vi "update_counter_entry_small.vi"(8 "error in":errorcluster, 10 "Integer Time":i64, 11 "input cluster":cluster{"data":u32, "data":u32}) -> (0 "error out":errorcluster)   [LabVIEW 2013]
doc: "Creates a new row in the counter or counter_small table."
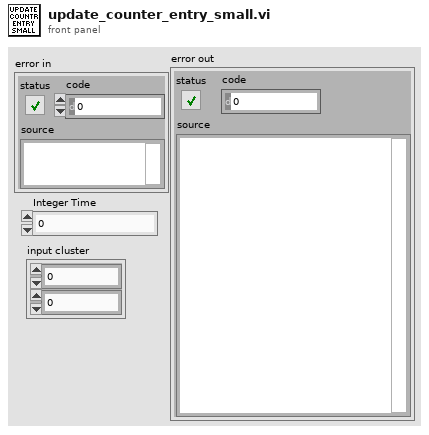
[diagram p1: front panel]
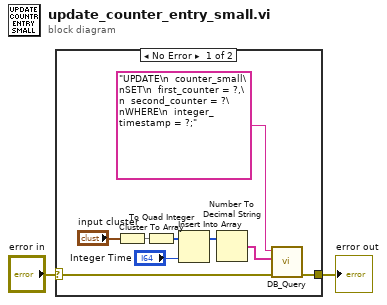
[diagram p0: block diagram]
diagram:
  n1 = case shown="No Error" "error in" {
    selector: "error in" -> [w10 w12]
    tunnel: [w11 w12] -> w1
    frame No Error {
      n2 = Cluster To Array(cluster="input cluster") -> (array=w7:u32[])
      n3 = To Quad Integer(1:w7) -> (0:w3:i64[])
      n4 = Insert Into Array(array=w3, new element="Integer Time") -> (w6:i64[])  [unwired: 1 in]
      n5 = Number To Decimal String(number=w6) -> (decimal integer string=w4:string[])  [unwired: 1 in]
      n6 = call "DB_Query.vi"("error in (no error)"=w10, "Parameters"=w4, "Parameterized Query"="UPDATE\n  counter_small\nSET\n  first_counter = ?,\n  second_counter = ?\nWHERE\n  integer_timestamp = ?;") -> ("error out"=w11:errorcluster)  [unwired: 6 in, 2 out]
    }
    frame Error {
    }
  }
  "error out" <- w1
